vi "新写入SN.vi"(0 "日期":string, 7 "流水号":string, 11 "error in":errorcluster) -> (6 "return":i32, 15 "error out":errorcluster)   [LabVIEW 2016]
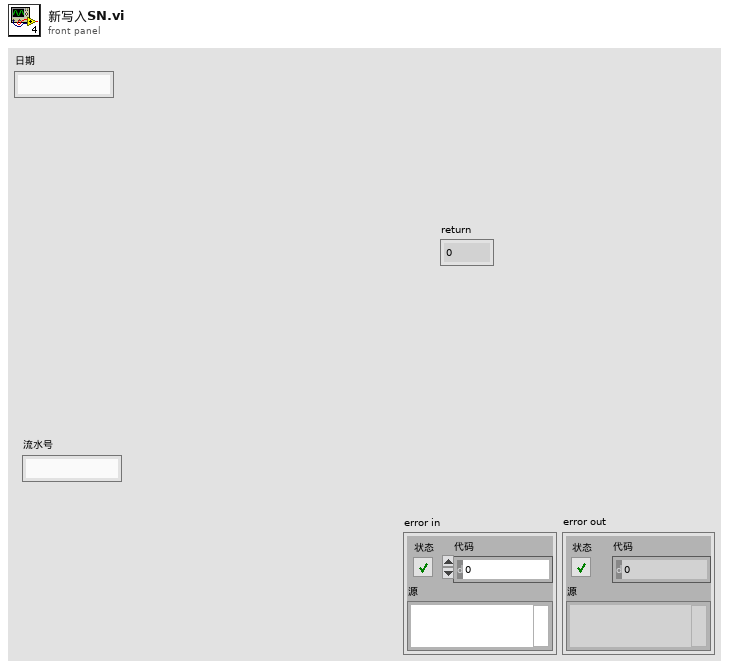
[diagram p1: front panel]
types:
  T1 = cluster{"byCmdType":u8, "bySubCmd":u8, "byPara":u8, "byAddr_h":u8, "byAddr_l":u8, "byAddr_ll":u8, "byLen_h":u8, "byLen_l":u8}
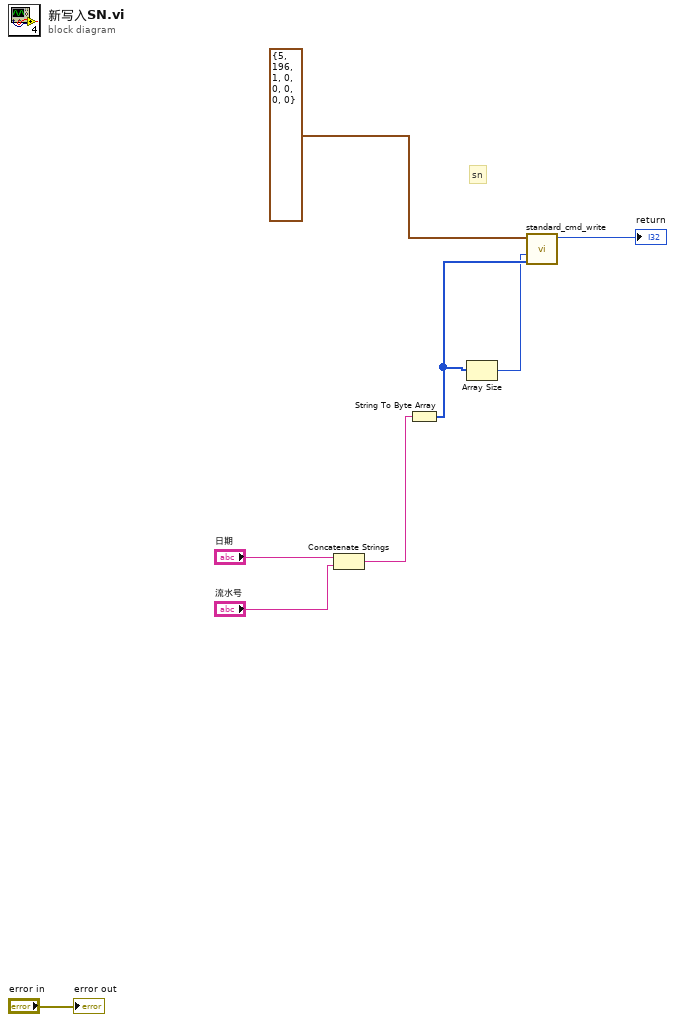
[diagram p0: block diagram]
diagram:
  # "sn"
  n1 = Concatenate Strings("日期", "流水号") -> (w7:string)
  n2 = String To Byte Array(string=w7) -> (unsigned byte array=w6:u8[])
  n3 = Array Size(array=w6) -> (size(s)=w5:i32)
  n4 = call "standard_cmd_write.vi"("data"=w6, "dwLen"=w5, "cmd_std_header_t"=T1 {"byCmdType"=5, "bySubCmd"=196, "byPara"=1, "byAddr_h"=0, "byAddr_l"=0, "byAddr_ll"=0, "byLen_h"=0, "byLen_l"=0}) -> ("return"=→"return":i32)  [unwired: 7 in, 1 out]
  "error out" <- "error in"
